vi "Finalize Hardware.vi"(8 "error in":errorcluster, 11 "module reference":T1) -> (0 "error out":errorcluster)   [LabVIEW 2020, in "AIM MIL-STD-1553 Engine.lvlib" / "Implementation.lvlib" / "Shared Resources.lvclass"]
uses:
  Hardware API/Module Reference.ctl
  Implementation/Shared Resources/Shared Resources.lvclass
  Hardware API/AIM MIL-STD-1553 Hardware API.lvlib
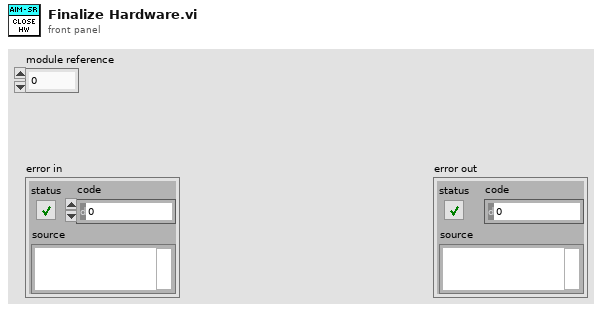
[diagram p1: front panel]
types:
  T1 = typedef "AIM MIL-STD-1553 Hardware API.lvlib/Module Reference.ctl" = u32
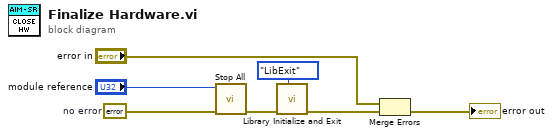
[diagram p0: block diagram]
diagram:
  w5 = errorcluster {"status"=FALSE, "code"=0, "source"=""}  # no error
  n1 = call "Stop All.vi"("error in"=w5, "module handle"="module reference") -> ("error out"=w3:errorcluster)  [unwired: 8 in, 1 out]
  n2 = call "Library Initialize and Exit.vi"("action"=enum16{"LibInit", "LibExit"}."LibExit", "error in"=w3) -> ("error out"=w2:errorcluster)  [unwired: 8 in, 1 out]
  n3 = Merge Errors("error in", w2) -> (→"error out":errorcluster)
